vi "Get Joint Position.vi"(6 "JointType":T1, 8 "error in (no error)":errorcluster, 10 "Joints":refnum<k24>, 11 "KinectSensor Reference":refnum<k24>) -> (0 "error out":errorcluster, 2 "Joints out":refnum<k24>, 3 "Joint Position":T2)   [LabVIEW 2011, in "KinectOne.lvlib"]
uses:
  KinectOne.lvlib
  Microsoft.Kinect
  Type Defs/Joint Position.ctl
  Type Defs/JointType.ctl
  Constants.vi
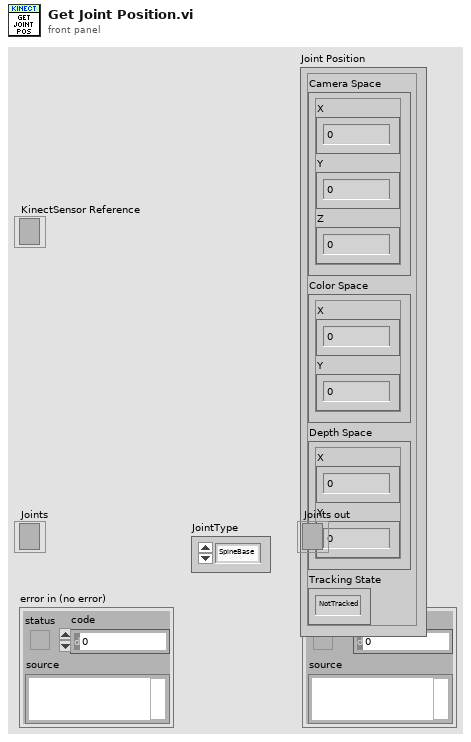
[diagram p1: front panel]
types:
  T1 = typedef "KinectOne.lvlib/JointType.ctl" = enum16{"SpineBase", "SpineMid", "Neck", "Head", "ShoulderLeft", "ElbowLeft", "WristLeft", "HandLeft", "ShoulderRight", "ElbowRight", "WristRight", "HandRight", "HipLeft", "KneeLeft", "AnkleLeft", "FootLeft", "HipRight", "KneeRight", "AnkleRight", "FootRight", "SpineShoulder", "HandTipLeft", "ThumbLeft", "HandTipRight", "ThumbRight"}
  T2 = typedef "KinectOne.lvlib/Joint Position.ctl" = cluster{"Camera Space":cluster{"X":dbl, "Y":dbl, "Z":dbl}, "Color Space":cluster{"X":dbl, "Y":dbl}, "Depth Space":cluster{"X":dbl, "Y":dbl}, "Tracking State":enum16{"NotTracked", "Inferred", "Tracked"}}
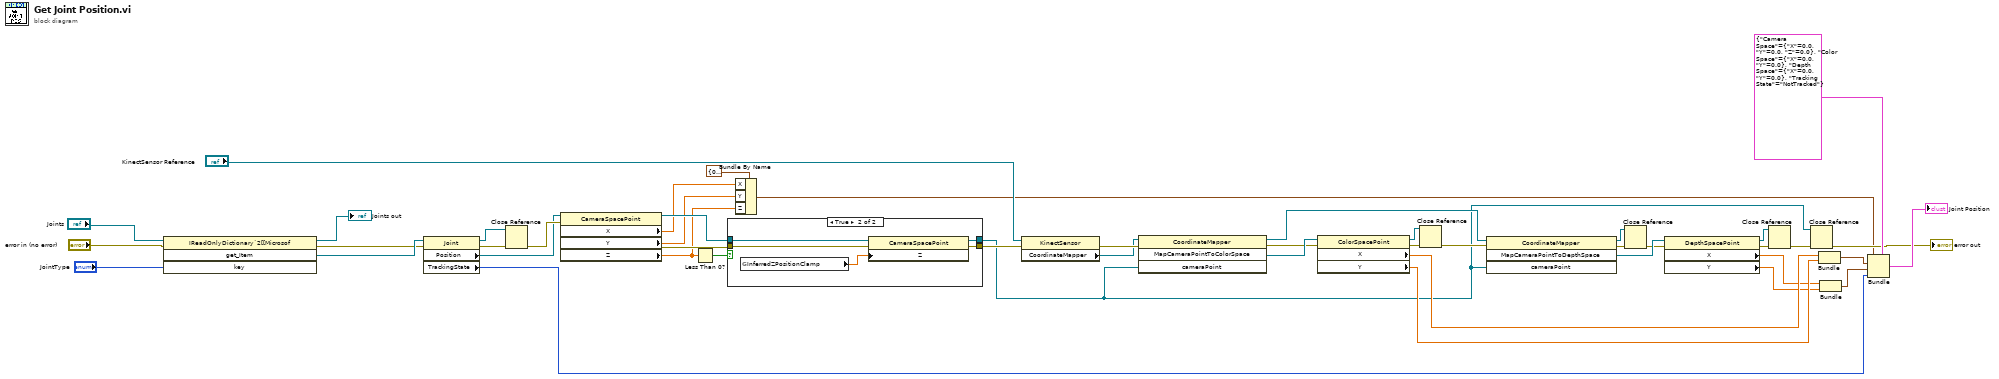
[diagram p0: block diagram]
diagram:
  n1 = invoke class="IReadOnlyDictionary`2[[Microsof" method="get_Item"(reference="Joints", error in="error in (no error)", "key"="JointType") -> (reference out=→"Joints out":refnum<k24>, error out=w29:errorcluster, "get_Item"=w36:refnum<k24>)  [unwired: 1 in, 1 out]
  n2 = property class="Joint"(reference=w36, error in=w29) -> (reference out=w33:refnum<k24>, error out=w34:errorcluster, "Position"=w1:refnum<k24>, "TrackingState"=w9:i32)
  n3 = Close Reference(reference=w33, error in (no error)=w34) -> (error out=w32:errorcluster)
  n4 = property class="CameraSpacePoint"(reference=w1, error in=w32) -> (reference out=w42:refnum<k24>, error out=w41:errorcluster, "X"=w5:sgl, "Y"=w4:sgl, "Z"=w3:sgl)
  n5 = Less Than 0?(x=w3) -> (x < 0?=w43:bool)
  n6 = case shown="True" w43 {
    tunnel: w42 -> [w47 w52]
    tunnel: w41 -> [w48 w51]
    tunnel: [w48 w50] -> w40
    tunnel: [w47 w49] -> w11
    frame False {
    }
    frame True {
      n7 = global read "Constants.vi" "InferredZPositionClamp"() -> (w53:sgl)
      n8 = property class="CameraSpacePoint"(reference=w52, error in=w51, "Z"=w53) -> (reference out=w49:refnum<k24>, error out=w50:errorcluster)
    }
  }
  n9 = Bundle By Name(cluster=cluster{"X":sgl, "Y":sgl, "Z":sgl} {"X"=0.0, "Y"=0.0, "Z"=0.0} ("Camera Space"), "X"=w5, "Y"=w4, "Z"=w3) -> (w2:cluster{"X":sgl, "Y":sgl, "Z":sgl})
  n10 = property class="KinectSensor"(reference="KinectSensor Reference", error in=w40) -> (error out=w46:errorcluster, "CoordinateMapper"=w45:refnum<k24>)  [unwired: 1 out]
  n11 = invoke class="CoordinateMapper" method="MapCameraPointToColorSpace"(reference=w45, error in=w46, "cameraPoint"=w11) -> (reference out=w17:refnum<k24>, error out=w18:errorcluster, "MapCameraPointToColorSpace"=w27:refnum<k24>)  [unwired: 1 in, 1 out]
  n12 = property class="ColorSpacePoint"(reference=w27, error in=w18) -> (reference out=w25:refnum<k24>, error out=w26:errorcluster, "X"=w38:sgl, "Y"=w39:sgl)
  n13 = Close Reference(reference=w25, error in (no error)=w26) -> (error out=w13:errorcluster)
  n14 = invoke class="CoordinateMapper" method="MapCameraPointToDepthSpace"(reference=w17, error in=w13, "cameraPoint"=w11) -> (reference out=w21:refnum<k24>, error out=w23:errorcluster, "MapCameraPointToDepthSpace"=w24:refnum<k24>)  [unwired: 1 in, 1 out]
  n15 = Close Reference(reference=w21, error in (no error)=w23) -> (error out=w22:errorcluster)
  n16 = property class="DepthSpacePoint"(reference=w24, error in=w22) -> (reference out=w19:refnum<k24>, error out=w20:errorcluster, "X"=w16:sgl, "Y"=w15:sgl)
  n17 = Close Reference(reference=w19, error in (no error)=w20) -> (error out=w14:errorcluster)
  n18 = Close Reference(reference=w11, error in (no error)=w14) -> (error out=→"error out":errorcluster)
  n19 = Bundle("X"=w38, "Y"=w39) -> (w7:cluster{"X":sgl, "Y":sgl})  [unwired: 1 in]
  n20 = Bundle("X"=w16, "Y"=w15) -> (w8:cluster{"X":sgl, "Y":sgl})  [unwired: 1 in]
  n21 = Bundle(cluster=T2 {"Camera Space"={"X"=0.0, "Y"=0.0, "Z"=0.0}, "Color Space"={"X"=0.0, "Y"=0.0}, "Depth Space"={"X"=0.0, "Y"=0.0}, "Tracking State"=enum."NotTracked"} ("Joint Position"), "Camera Space"=w2, "Color Space"=w7, "Depth Space"=w8, "Tracking State"=w9) -> (→"Joint Position":T2)
